vi "find owning target.vi"(8 "error in":errorcluster, 11 "node":refnum<data-value>) -> (0 "error out":errorcluster, 2 "target configuration":refnum<class "PL_Target Configuration.lvclass">, 3 "target":refnum<data-value>)   [LabVIEW 2013, in "TEC editor node.lvclass"]
uses:
  TEC editor node.lvclass
  <vilib>/NI/DCAF/Tag Editor Core/Configuration Editor/Classes/Targets/Targets.lvclass
  <vilib>/NI/Configuration Framework/Node/NISE_CEF_Node.lvclass
  <vilib>/NI/DCAF/Tag Editor Core/Framework Configuration Classes/target configuration/PL_Target Configuration.lvclass
  <vilib>/NI/DCAF/Tag Editor Core/Configuration Editor/Classes/Targets/read target configuration.vi
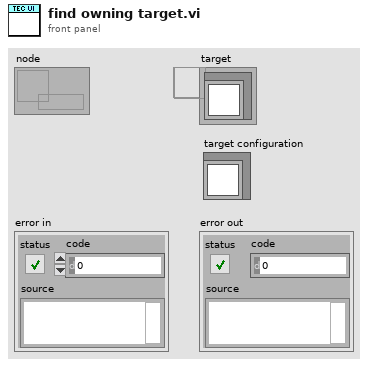
[diagram p1: front panel]
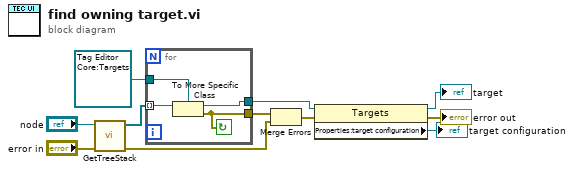
[diagram p0: block diagram]
diagram:
  n1 = call <vilib>:"GetTreeStack.vi"("error in"="error in", "node in"="node") -> ("error out"=w9:errorcluster, "parents"=w6:refnum<data-value>[])  [unwired: 8 in]
  n2 = for {
    tunnel: w6 -> [w15] mode=indexing
    tunnel: [w14] -> w5
    tunnel: refnum<data-value> refnum ("node in") -> [w13]
    tunnel: [w12] -> w8
    stop <- w12 continue-if-true
    n3 = To More Specific Class(target class=w13, reference=w15) -> (specific class reference=w14:refnum<data-value>, error out=w12:errorcluster)  [unwired: 1 in]
  }
  n4 = Merge Errors(w8, w9) -> (w3:errorcluster)
  n5 = property class="Targets"(reference=w5, error in=w3) -> (reference out=→"target":refnum<data-value>, error out=→"error out":errorcluster, "Properties:target configuration"=→"target configuration":refnum<class "PL_Target Configuration.lvclass">)
